vi "Test4He.vi"() -> ()   [LabVIEW 2018]
panel:
  out "4He Gauge Error":errorcluster={"status"=TRUE, "code"=-1073807343, "source"="VISA Open in Turbulence.vi"}
  in  "stop":bool
  out "Pressure":dbl
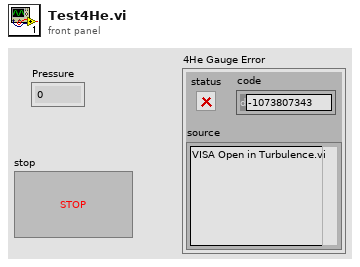
[diagram p1: front panel]
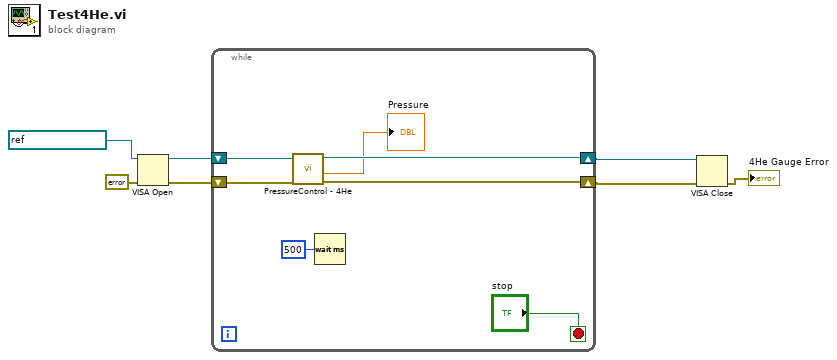
[diagram p0: block diagram]
diagram:
  n1 = VISA Open(error in (no error)=errorcluster {"status"=FALSE, "code"=0, "source"=""}, VISA resource name=refnum<visa-resource-name> "TankPressure" ("Pressure Gauge")) -> (VISA resource name=w5:refnum<visa-resource-name>, error out=w4:errorcluster)  [unwired: 3 in]
  n2 = while {
    shift-right: [w11] -> w2
    shift-left: w4 -> [w14]
    shift-right: [w12] -> w1
    shift-left: w5 -> [w13]
    stop <- "stop" stop-if-true
    n3 = call "PressureControl - 4He.vi"("error in (no error)"=w14, "VISA resource name"=w13) -> ("error out"=w11:errorcluster, "Pressure"=→"Pressure":dbl, "VISA resource name out"=w12:refnum<visa-resource-name>)  [unwired: 6 in, 1 out]
    n4 = Wait (ms)(milliseconds to wait=u32 500) -> ()  [unwired: 1 out]
  }
  n5 = VISA Close(VISA resource name=w1, error in (no error)=w2) -> (error out=→"4He Gauge Error":errorcluster)
